vi "Measurement Logic.vi"() -> ()   [LabVIEW 2021, in "NIDCPowerSourceDCVoltage.lvlib"]
uses:
  NIDCPowerSourceDCVoltage.lvlib
  Measurement Configuration.ctl
  Measurement Results.ctl
  <vilib>/Plug-In SDKs/Measurements/Measure Call Context/Measure Call Context.lvclass
  Json Logger Client/Json Logger Client.lvclass
  <vilib>/Plug-In SDKs/Clients/Session Management V1/Session Reservation/Session Reservation.lvclass
  <vilib>/Plug-In SDKs/Sessions/niDCPower/NI Session Management niDCPower.lvlib
panel:
  in  "error in":errorcluster
  out "error out":errorcluster
  out "measure call context out":refnum<class "Measure Call Context.lvclass">
  in  "measure call context in":refnum<class "Measure Call Context.lvclass">
  out "measurement results":T1
  in  "measurement configuration":T2={"pin_names"=[], "voltage_level"=6.0, "voltage_level_range"=6.0, "current_limit"=0.01, "current_limit_range"=0.01, "source_delay"=0.0}
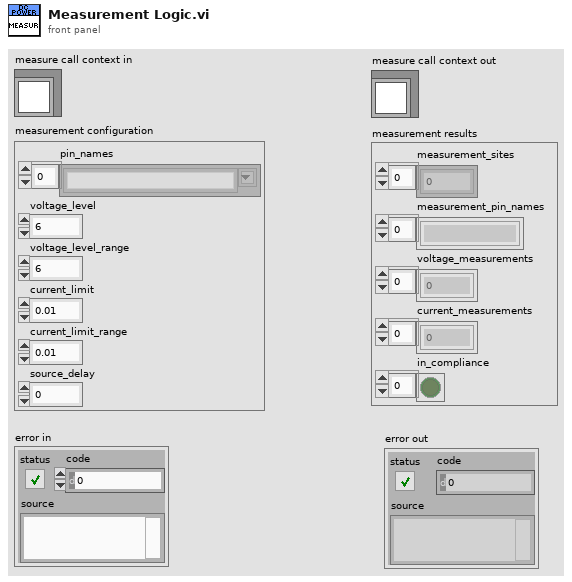
[diagram p1: front panel]
types:
  T1 = typedef "NIDCPowerSourceDCVoltage.lvlib/Measurement Results.ctl" = cluster{"measurement_sites":i32[], "measurement_pin_names":string[], "voltage_measurements":dbl[], "current_measurements":dbl[], "in_compliance":bool[]}
  T2 = typedef "NIDCPowerSourceDCVoltage.lvlib/Measurement Configuration.ctl" = cluster{"pin_names":string[], "voltage_level":dbl, "voltage_level_range":dbl, "current_limit":dbl, "current_limit_range":dbl, "source_delay":dbl}
  T3 = typedef "NI Session Management niDCPower.lvlib/Connection with Session.ctl" = cluster{"connection":T4, "session":refnum<k15>}
  T4 = typedef "NI Session Management V1 Client.lvlib/Session Reservation.lvclass/Connection.ctl" = cluster{"pin or relay name":string, "site":i32, "instrument type id":string, "channel":string}
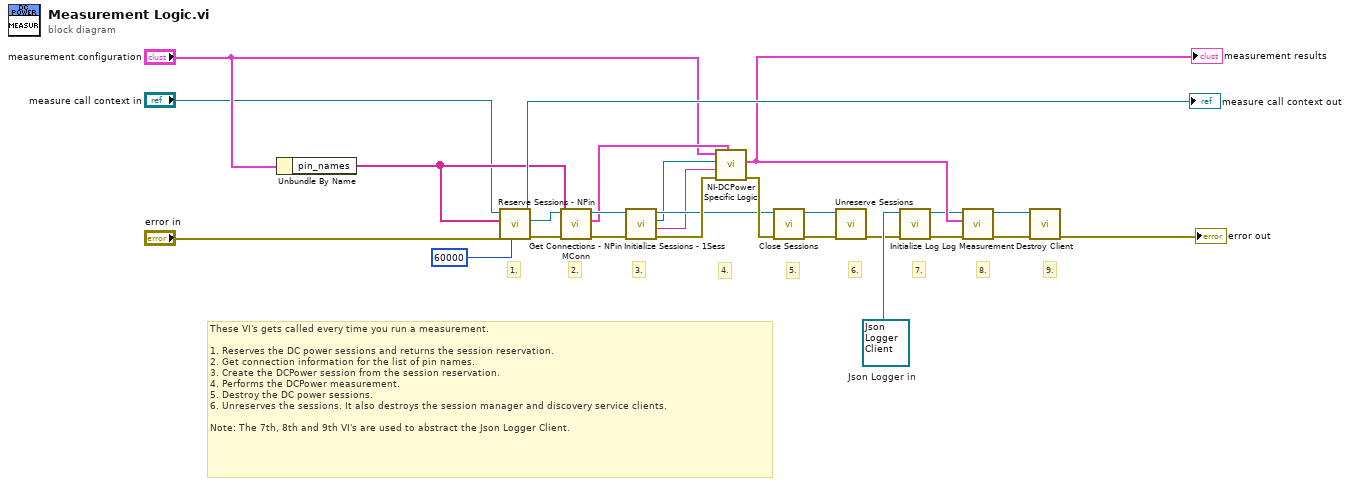
[diagram p0: block diagram]
diagram:
  w10 = refnum<class "Json Logger Client.lvclass"> refnum  # Json Logger in
  # "9."
  # "8."
  # "7."
  # "6."
  # "These VI's gets called every time you run a measurement.\n\n1. Reserves the DC power sessions and returns the session reservation.\n2. Get connection information for the list of pin names.\n3. Create the DCPower session from the session reservation.\n4. Performs the DCPower measurement.\n5. Destroy the DC power sessions.\n6. Unreserves the sessions. It also destroys the session manager and discovery service clients.\n\nNote: The 7th, 8th and 9th VI's are used to abstract the Json Logger Client."
  # "5."
  # "4."
  # "3."
  # "2."
  # "1."
  n1 = Unbundle By Name("measurement configuration") -> ("pin_names"=w16:string[])
  n2 = call <vilib>:"Reserve Sessions - NPin.vi"("timeout (ms)"=60000, "error in"="error in", "pin or relay names"=w16, "measurement context in"="measure call context in") -> ("error out"=w19:errorcluster, "session reservation out"=w17:refnum<class "Session Reservation.lvclass">, "measurement context out"=→"measure call context out":refnum<class "Measure Call Context.lvclass">)  [unwired: 5 in]
  n3 = call <vilib>:"Get Connections - NPin MConn.vi"("error in"=w19, "pin or relay names"=w16, "session reservation in"=w17) -> ("error out"=w18:errorcluster, "connections"=w14:T3[], "session reservation out"=w15:refnum<class "Session Reservation.lvclass">)  [unwired: 6 in]
  n4 = call <vilib>:"Initialize Sessions - 1Sess.vi"("error in"=w18, "session reservation in"=w15) -> ("error out"=w26:errorcluster, "channel list"=w12:string, "session"=w13:refnum<k15>, "session reservation out"=w22:refnum<class "Session Reservation.lvclass">)  [unwired: 6 in]
  n5 = call "NI-DCPower Specific Logic.vi"("connections"=w14, "error in"=w26, "channel list"=w12, "instrument handle"=w13, "Measurement Configuration"="measurement configuration") -> ("error out"=w25:errorcluster, "Measurement Results"=w8:T1)  [unwired: 4 in, 1 out]
  "measurement results" <- w8
  n6 = call <vilib>:"Close Sessions.vi"("error in"=w25, "session reservation in"=w22) -> ("error out"=w24:errorcluster, "session reservation out"=w23:refnum<class "Session Reservation.lvclass">)  [unwired: 8 in]
  n7 = call <vilib>:"Unreserve Sessions.vi"("error in"=w24, "session reservation in"=w23) -> ("error out"=w3:errorcluster)  [unwired: 9 in]
  n8 = call-dynamic "Initialize Log.vi"("error in (no error)"=w3, "Json Logger in"=w10) -> ("error out"=w9:errorcluster, "Json Logger out"=w7:refnum<class "Json Logger Client.lvclass">)  [unwired: 8 in]
  n9 = call-dynamic "Log Measurement.vi"("error in (no error)"=w9, "Measurement Results"=w8, "Json Logger in"=w7) -> ("error out"=w5:errorcluster, "Json Logger out"=w6:refnum<class "Json Logger Client.lvclass">)  [unwired: 7 in]
  n10 = call-dynamic "Destroy Client.vi"("error in (no error)"=w5, "Json Logger in"=w6) -> ("error out"=→"error out":errorcluster)  [unwired: 8 in, 1 out]
